vi "picoscopeWriteChannelToTDMS.vi"(4 "index":i32, 6 "EnableChA":T1, 7 "ScopeTraces":waveform(dbl)[](array[waveform]), 8 "error in (no error)":errorcluster, 9 "channel name":string, 10 "group name in (Untitled)":string="pico", 11 "tdms file":refnum<k34>) -> (0 "error out":errorcluster, 2 "group name out":string, 3 "Refnum out":refnum<k34>)   [LabVIEW 2020, in "PicoscopeV2.lvclass"]
uses:
  PicoscopeV2.lvclass
  shared/OnOffTypeDef.ctl
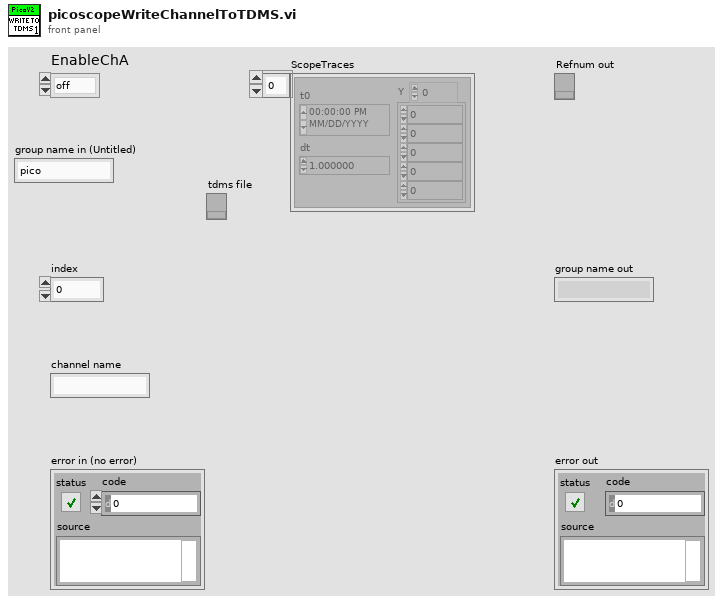
[diagram p1: front panel]
types:
  T1 = typedef "OnOffTypeDef.ctl" = enum16{"off", "on"}
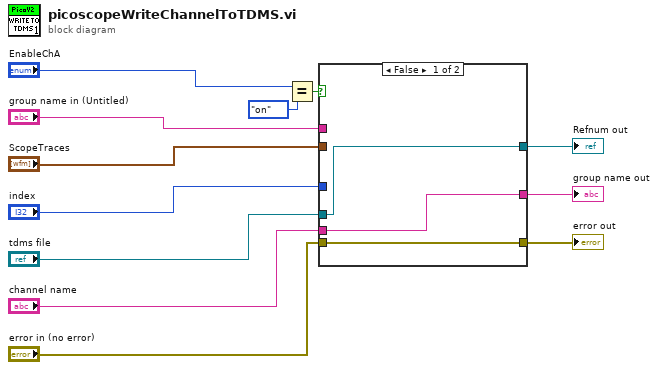
[diagram p0: block diagram]
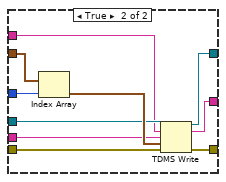
[diagram p2: hidden frame]
diagram:
  n1 = Equal?(x="EnableChA", y=OnOffTypeDef."on") -> (x = y?=w6:bool)
  n2 = case shown="False" w6 {
    tunnel: "ScopeTraces" -> [_ w25]
    tunnel: [w14 w23] -> w8
    tunnel: [w13 w22] -> w9
    tunnel: [w15 w21] -> w10
    tunnel: "error in (no error)" -> [w15 w19]
    tunnel: "index" -> [_ w20]
    tunnel: "tdms file" -> [w14 w18]
    tunnel: "group name in (Untitled)" -> [_ w17]
    tunnel: "channel name" -> [w13 w16]
    frame False {
    }
    frame True {
      n3 = Index Array(array=w25, index=w20) -> (element=w24:waveform(dbl))
      n4 = TDMS Write(0:w18, 5:w17, 7:w16, 9:w24, 11:w19) -> (4:w23:refnum<k34>, 6:w22:string, 15:w21:errorcluster)  [unwired: 1 in, 1 out]
    }
  }
  "error out" <- w10
  "group name out" <- w9
  "Refnum out" <- w8
